vi "read single axis Field Module.vi"(0 "Magnet Device Select":string(combo)="Elsa Magnet", 5 "error in (no error)":errorcluster, 7 "Init":bool, 9 "Exec":bool, 11 "final":bool) -> (14 "FIeld mT":dbl format="%_9f", 19 "error out":errorcluster)   [LabVIEW 2024]
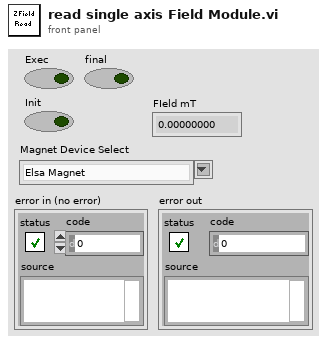
[diagram p1: front panel]
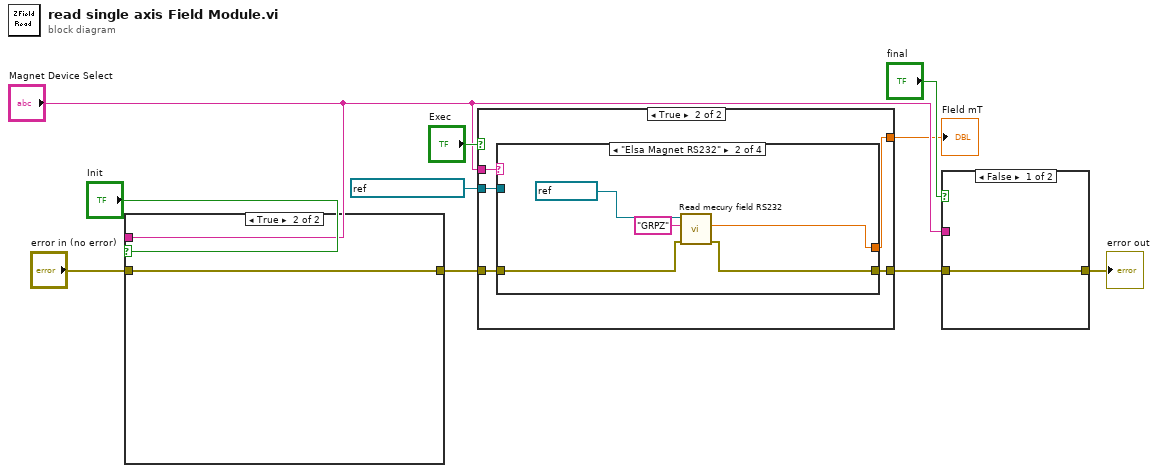
[diagram p0: block diagram]
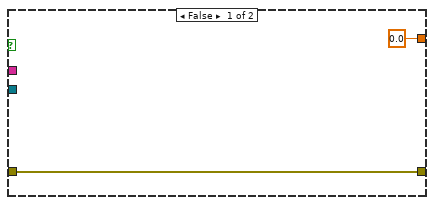
[diagram p6: hidden frame]
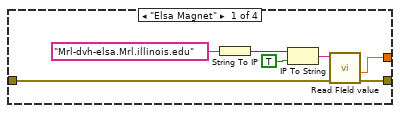
[diagram p7: hidden frame]
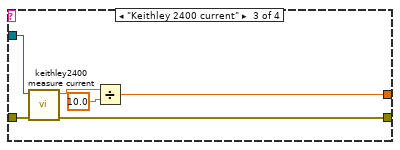
[diagram p8: hidden frame]
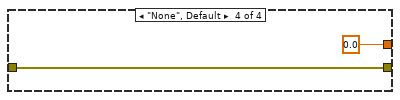
[diagram p9: hidden frame]
diagram:
  n1 = case shown="True" "Init" {
    tunnel: "error in (no error)" -> [w11 w12]
    tunnel: [w11 w12] -> w7
    tunnel: "Magnet Device Select" -> [_ _]
    frame False {
    }
    frame True {
    }
  }
  n2 = case shown="True" "Exec" {
    tunnel: w7 -> [w14 w19]
    tunnel: [w14 w16] -> w5
    tunnel: "Magnet Device Select" -> [_ w18]
    tunnel: refnum<visa-resource-name> "GPIB0::22::INSTR" ("VISA resource name") -> [_ w17]
    tunnel: [0.0 ("Z FIeld mT") w15] -> w1
    frame False {
    }
    frame True {
      n3 = case shown="\"Elsa Magnet RS232\"" w18 {
        tunnel: w19 -> [w26 w31 w37 w39]
        tunnel: w17 -> [_ _ w35 _]
        tunnel: [w25 w30 w36 w39] -> w16
        tunnel: [w24 w29 w33 0.0 ("Z FIeld mT")] -> w15
        frame "Elsa Magnet" {
          n4 = String To IP(1:"Mrl-dvh-elsa.Mrl.illinois.edu" ("IP Address")) -> (0:w22:u32)
          n5 = IP To String(1:TRUE ("dot notation? (F)"), 2:w22) -> (0:w21:string)
          n6 = call "Read FIeld value.vi"("error in (no error)"=w26, "IP Address"=w21) -> ("error out"=w25:errorcluster, "Z FIeld mT"=w24:dbl)  [unwired: 6 in, 2 out]
        }
        frame "Elsa Magnet RS232" {
          n7 = call "Read mecury field RS232.vi"("error in (no error)"=w31, "Device on PSU"="GRPZ", "VISA resource name"=refnum<visa-resource-name> "COM1") -> ("error out"=w30:errorcluster, "FIeld mT"=w29:dbl)  [unwired: 6 in, 1 out]
        }
        frame "Keithley 2400 current" {
          n8 = call "keithley2400 measure current.vi"("error in (no error)"=w37, "VISA resource name"=w35) -> ("error out"=w36:errorcluster, "Current mA"=w34:dbl)  [unwired: 8 in]
          n9 = Divide(x=w34, y=10.0) -> (x/y=w33:dbl)
        }
        frame "None", Default {
        }
      }
    }
  }
  "FIeld mT" <- w1
  n10 = case shown="False" "final" {
    tunnel: w5 -> [w40 w43]
    tunnel: [w40 w42] -> w4
    tunnel: "Magnet Device Select" -> [_ w41]
    frame False {
    }
    frame True {
      n11 = case shown="\"Keithley 2400 current\"" w41 {
        tunnel: w43 -> [w44 w45 w46]
        tunnel: [w44 w45 w46] -> w42
        frame "Elsa Magnet" {
        }
        frame "Keithley 2400 current" {
        }
        frame "None", Default {
        }
      }
    }
  }
  "error out" <- w4
